vi "修改属性.vi"(6 "属性名称":string, 8 "错误输入（无错误）":errorcluster, 9 "属性值":variant, 10 "测试时间":timestamp, 11 "db file":path) -> (0 "错误输出":errorcluster)   [LabVIEW 2020]
uses:
  <vilib>/drjdpowell/SQLite Library/SQL Connection/Connection.lvclass
  <vilib>/drjdpowell/SQLite Library/SQL Connection/Open (path).vi
  <vilib>/drjdpowell/SQLite Library/SQL Statement/SQL Statement.lvclass
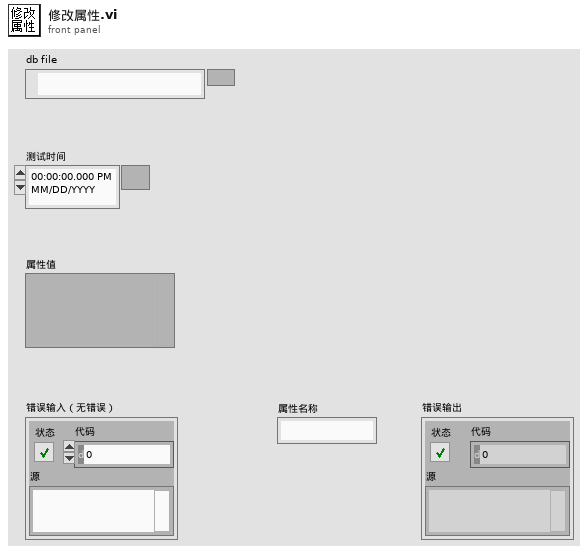
[diagram p1: front panel]
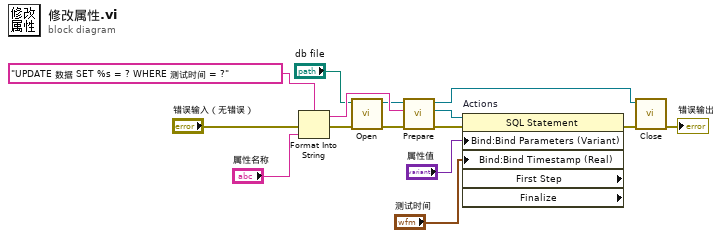
[diagram p0: block diagram]
diagram:
  n1 = Format Into String(format string="UPDATE 数据 SET %s = ? WHERE 测试时间 = ?", error in="错误输入（无错误）", "属性名称") -> (resulting string=w11:string, error out=w10:errorcluster)  [unwired: 1 in]
  n2 = call-poly <vilib>:"Open.vi"("error in (no error)"=w10, "db file"="db file") -> ("error out"=w9:errorcluster, "SQLite Connection"=w8:refnum<class "Connection.lvclass">)  [unwired: 8 in]
  n3 = call <vilib>:"Prepare.vi"("error in (no error)"=w9, "SQL"=w11, "SQLite Connection in"=w8) -> ("error out"=w15:errorcluster, "SQL Statement"=w14:refnum<class "SQL Statement.lvclass">, "SQLite Connection"=w5:refnum<class "Connection.lvclass">)  [unwired: 4 in, 2 out]
  n4 = property on="Actions" class="SQL Statement" props=["Bind:Bind Parameters (Variant)", "Bind:Bind Timestamp (Real)", "First Step", "Finalize"](reference=w14, error in=w15, "Bind:Bind Parameters (Variant)"="属性值", "Bind:Bind Timestamp (Real)"="测试时间") -> (error out=w6:errorcluster)  [unwired: 3 out]
  n5 = call-dynamic "Close.vi"("error in (no error)"=w6, "SQLite Connection in"=w5) -> ("error out"=→"错误输出":errorcluster)  [unwired: 9 in]
